vi "SearchFolder_OfAFile.vi"(0 "Folder_Mgmt out":refnum<class "Folder_Mgmt.lvclass">, 2 "FileToSearch":string, 3 "error in (no error)":errorcluster) -> (7 "Folder_Mgmt out 2":refnum<class "Folder_Mgmt.lvclass">, 9 "FolderOfFile":string, 10 "error out":errorcluster)   [LabVIEW 2016, in "Folder_Mgmt.lvclass"]
uses:
  Folder_Mgmt.lvclass
  Folder_Mgmt.lvclass/Folder_Mgmt.ctl
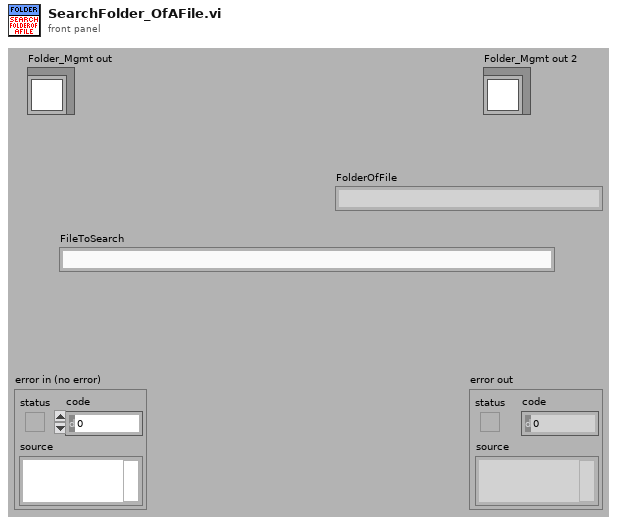
[diagram p1: front panel]
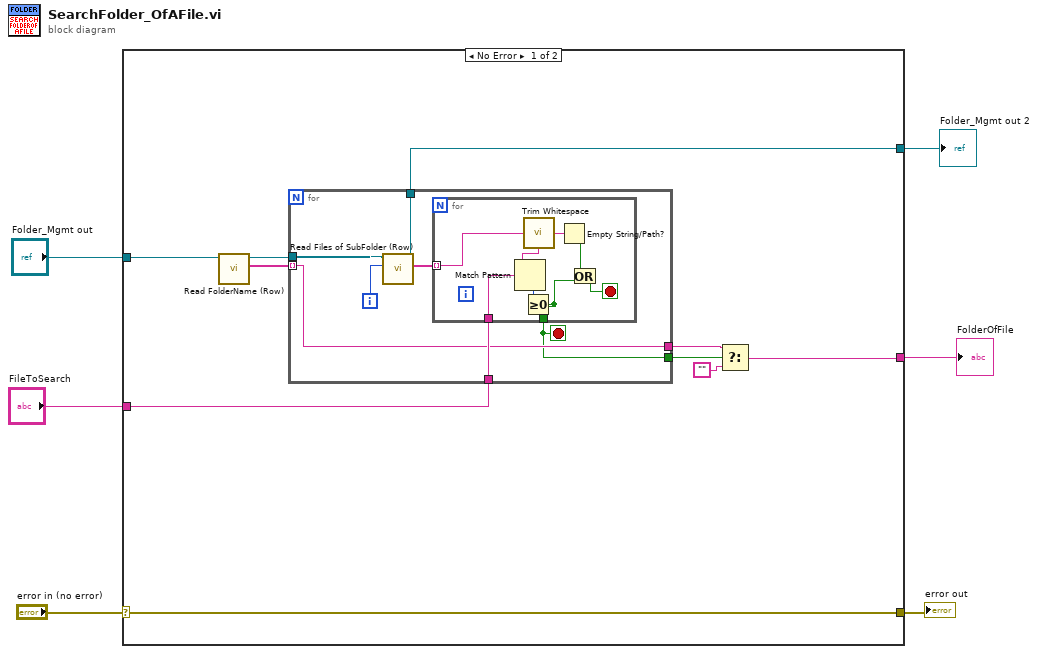
[diagram p0: block diagram]
diagram:
  n1 = case shown="No Error" "error in (no error)" {
    selector: "error in (no error)" -> [w16 w32]
    tunnel: [w16 w32] -> w5
    tunnel: "Folder_Mgmt out" -> [w14 w31]
    tunnel: "FileToSearch" -> [w15 _]
    tunnel: [w11 _] -> w2
    tunnel: [w7 w31] -> w1
    frame No Error {
      n2 = call "Read FolderName (Row).vi"("Folder_Mgmt in"=w14) -> ("FolderName (Row)"=w12:string[], "Folder_Mgmt out"=w13:refnum<class "Folder_Mgmt.lvclass">)  [unwired: 8 in, 1 out]
      n3 = for {
        tunnel: w15 -> [w23]
        tunnel: w13 -> [w22]
        tunnel: w12 -> [w20] mode=indexing
        tunnel: [w20] -> w10
        tunnel: [w18] -> w9
        tunnel: [w17] -> w7
        i -> [w21]
        stop <- w18 stop-if-true
        n4 = call "Read Files of SubFolder (Row).vi"("RowIndex"=w21, "Folder_Mgmt in"=w22) -> ("FolderFiles (Row)"=w19:string[], "Folder_Mgmt out"=w17:refnum<class "Folder_Mgmt.lvclass">)  [unwired: 7 in, 1 out]
        n5 = for {
          tunnel: w23 -> [w29]
          tunnel: [w25] -> w18
          tunnel: w19 -> [w24] mode=indexing
          stop <- w26 stop-if-true
          n6 = call <vilib>:"Trim Whitespace.vi"("string"=w24) -> ("trimmed string"=w27:string)  [unwired: 1 in]
          n7 = Match Pattern(string=w27, regular expression=w29) -> (offset past match=w28:i32)  [unwired: 1 in, 3 out]
          n8 = Greater Or Equal To 0?(x=w28) -> (x >= 0?=w25:bool)
          n9 = Empty String/Path?(string/path=w27) -> (empty?=w30:bool)
          n10 = Or(x=w30, y=w25) -> (x .or. y?=w26:bool)
        }
      }
      n11 = Select(t=w10, s=w9, f="") -> (s? t:f=w11:string)
    }
    frame Error {
    }
  }
  "error out" <- w5
  "FolderOfFile" <- w2
  "Folder_Mgmt out 2" <- w1
